vi "R1GetLoops.vi"(7 "LabVIEW Web Service Request":refnum<class "Web Request.lvclass">, 10 "cRIONo":i32=1, 11 "ReactorNo":i32=1) -> (3 "Output array":string[](array[string]))   [LabVIEW 2016]
uses:
  <vilib>/wsapi/Web Request.lvclass
  <resource>/objmgr/ni.var.rc
panel:
  # "Use the Web Service Request input terminal to call the VIs on the Web Services palette. Do not remove it from the connector pane unless you don't need access to the palette."
  # "Each additional control wired to the connector pane will be available as an input in the URL. To include an indicator in terminal-mode output (the default setting), it must also be wired to the connector pane."
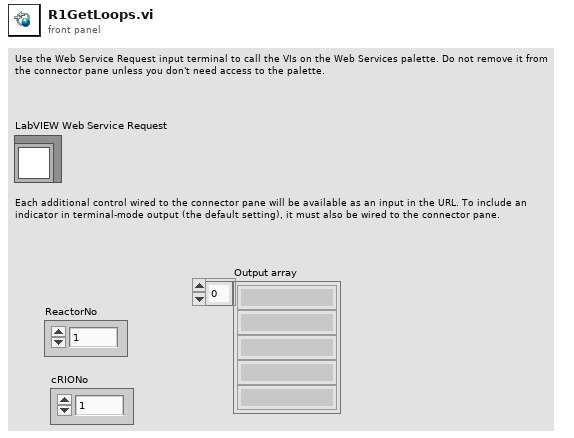
[diagram p1: front panel]
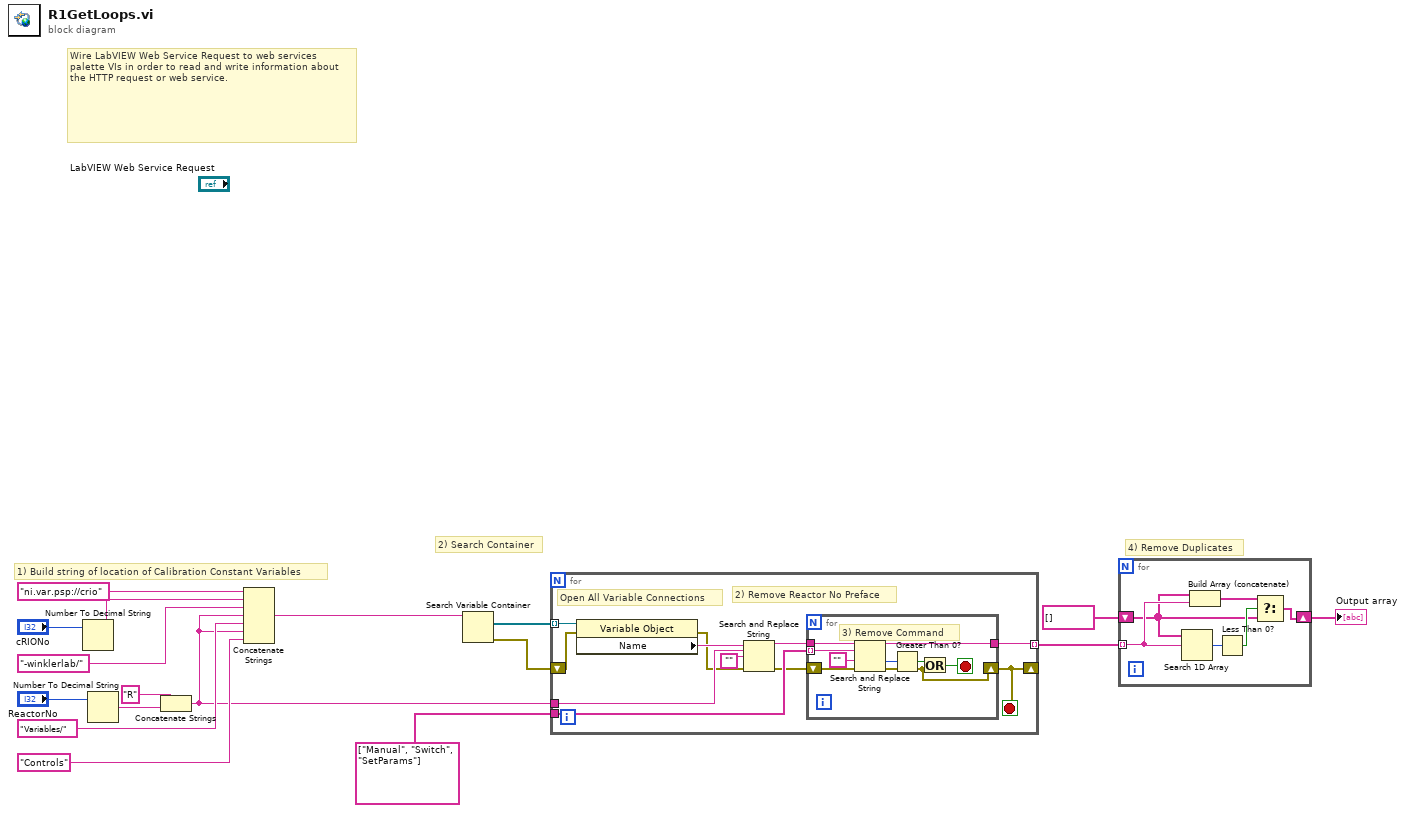
[diagram p0: block diagram]
diagram:
  # "4) Remove Duplicates"
  # "2) Search Container"
  # "1) Build string of location of Calibration Constant Variables"
  # "Wire LabVIEW Web Service Request to web services palette VIs in order to read and write information about the HTTP request or web service."
  n1 = Number To Decimal String(number="cRIONo") -> (decimal integer string=w12:string)  [unwired: 1 in]
  n2 = Number To Decimal String(number="ReactorNo") -> (decimal integer string=w15:string)  [unwired: 1 in]
  n3 = Concatenate Strings("R" ("string"), w15) -> (w5:string)
  n4 = Concatenate Strings("ni.var.psp://crio" ("string"), w12, "-winklerlab/" ("string"), w5, "Variables/" ("string"), w5, "Controls" ("string")) -> (w6:string)
  n5 = Search Variable Container(11:w6) -> (0:w9:errorcluster, 2:w8:refnum<k21>[])  [unwired: 5 in, 1 out]
  n6 = for {
    shift-right: [w19] -> _
    shift-left: w9 -> [w28]
    tunnel: w8 -> [w27] mode=indexing
    tunnel: w5 -> [w25]
    tunnel: string[] ["Manual", "Switch", "SetParams"] -> [w21]
    tunnel: [w18] -> w3 mode=indexing
    stop <- w19 stop-if-true
    # "2) Remove Reactor No Preface"
    # "Open All Variable Connections"
    n7 = property class="Variable Object"(reference=w27, error in=w28) -> (error out=w23:errorcluster, "Name"=w26:string)  [unwired: 1 out]
    n8 = Search and Replace String(input string=w26, search string=w25, replace string="", error in=w23) -> (result string=w22:string, error out=w20:errorcluster)  [unwired: 4 in, 2 out]
    n9 = for {
      tunnel: w22 -> [w37]
      tunnel: w21 -> [w36] mode=indexing
      shift-right: [w29] -> w19
      shift-left: w20 -> [w34]
      tunnel: [w33] -> w18
      stop <- w30 stop-if-true
      # "3) Remove Command"
      n10 = Search and Replace String(input string=w37, search string=w36, replace string="", error in=w34) -> (result string=w33:string, offset past replacement=w32:i32, error out=w29:errorcluster)  [unwired: 4 in, 1 out]
      n11 = Greater Than 0?(x=w32) -> (x > 0?=w31:bool)
      n12 = Or(x=w31, y=w29) -> (x .or. y?=w30:bool)
    }
  }
  n13 = for {
    tunnel: w3 -> [w43] mode=indexing
    shift-right: [w38] -> w1
    shift-left: string[] [] ("Output array 2") -> [w40]
    n14 = Search 1D Array(1D array=w40, element=w43) -> (index of element=w42:i32)  [unwired: 1 in]
    n15 = Build Array (concatenate)(w40, w43) -> (w39:string[])
    n16 = Less Than 0?(x=w42) -> (x < 0?=w41:bool)
    n17 = Select(t=w39, s=w41, f=w40) -> (s? t:f=w38:string[])
  }
  "Output array" <- w1
